vi "ADC.vi"(0 "Bits":i32, 5 "Channels":i32, 7 "Sampling rate":i32) -> (4 "Digital 1D":u8[](array[numeric]))   [LabVIEW 2020]
uses:
  <vilib>/numeric/Random Number (Range) DBL.vi
panel:
  out "Digital 2D":u8[][](array[numeric])
  out "unsigned byte array":u8[][](array[numeric])
  out "Error out":errorcluster
  in  "Error in":errorcluster
  out "Binary Array":string[](array[string])
  out "Digital Array":dbl[](array[numeric])
  out "Analog Array":dbl[](array[numeric])
  in  "Vref":dbl=5.0
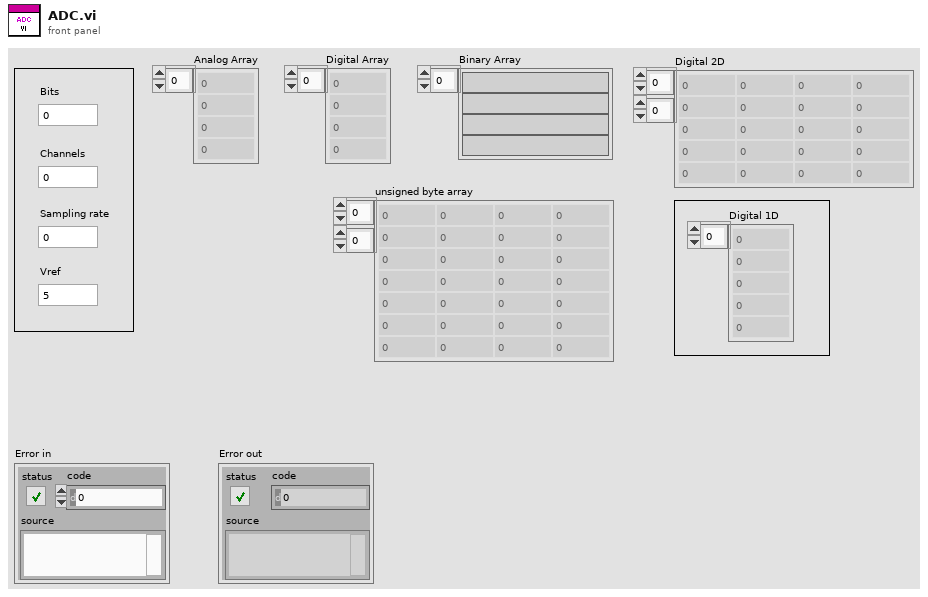
[diagram p1: front panel]
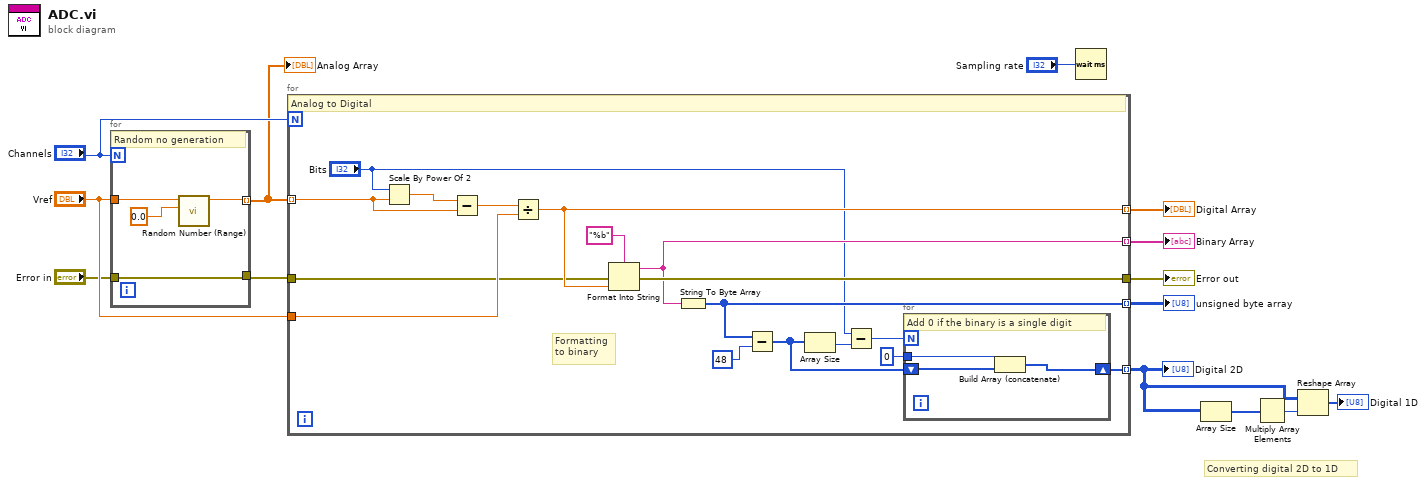
[diagram p0: block diagram]
diagram:
  # "Converting digital 2D to 1D"
  n1 = for {
    N: "Channels" -> [_]
    tunnel: "Vref" -> [w18]
    tunnel: [w16] -> w13 mode=indexing
    tunnel: "Error in" -> [w15]
    tunnel: [w15] -> w8
    # "Random no generation"
    n2 = call-poly <vilib>:"Random Number (Range).vi"("lower bound (0)"=0.0, "upper bound (100)"=w18) -> ("number"=w16:dbl)  [unwired: 9 in]
  }
  "Analog Array" <- w13
  n3 = for {
    N: "Channels" -> [_]
    tunnel: w13 -> [w34] mode=indexing
    tunnel: "Vref" -> [w32]
    tunnel: [w30] -> w11 mode=indexing
    tunnel: [w27] -> w7 mode=indexing
    tunnel: [w29] -> w10
    tunnel: w8 -> [w28]
    tunnel: [w26] -> w6 mode=indexing
    tunnel: [w19] -> w3 mode=indexing
    # "Formatting\nto binary"
    # "Analog to Digital"
    n4 = Scale By Power Of 2(n="Bits", x=w34) -> (x*2^n=w35:dbl)
    n5 = Subtract(x=w35, y=w34) -> (x-y=w33:dbl)
    n6 = Divide(x=w33, y=w32) -> (x/y=w30:dbl)
    n7 = Format Into String(format string="%b", error in=w28, w30) -> (resulting string=w27:string, error out=w29:errorcluster)  [unwired: 1 in]
    n8 = String To Byte Array(string=w27) -> (unsigned byte array=w26:u8[])
    n9 = Subtract(x=w26, y=u8 48) -> (x-y=w21:u8[])
    n10 = Array Size(array=w21) -> (size(s)=w24:i32)
    n11 = Subtract(x="Bits", y=w24) -> (x-y=w22:i32)
    n12 = for {
      N: w22 -> [_]
      shift-right: [w36] -> w19
      shift-left: w21 -> [w38]
      tunnel: u8 0 -> [w37]
      # "Add 0 if the binary is a single digit"
      n13 = Build Array (concatenate)(w37, w38) -> (w36:u8[])
    }
  }
  "Digital Array" <- w11
  "Binary Array" <- w7
  "Error out" <- w10
  "unsigned byte array" <- w6
  "Digital 2D" <- w3
  n14 = Wait (ms)(milliseconds to wait="Sampling rate") -> ()  [unwired: 1 out]
  n15 = Array Size(array=w3) -> (size(s)=w5:i32[])
  n16 = Multiply Array Elements(1:w5) -> (0:w4:i32)
  n17 = Reshape Array(w3, w4) -> (→"Digital 1D":u8[])
